vi "Example While Loop Some Operations 2.vi"(8 "Error In":errorcluster, 11 "Boolean":bool) -> (0 "Error Out":errorcluster, 3 "Numeric":i32)   [LabVIEW 2018]
doc: "Testing VI contains WhileLoop and som operations inside and some other constants and functions for numbers used inside WhileLoop. Just for example parsing."
uses:
  <vilib>/measure/NI_MABase.lvlib
panel:
  out "signal out 4":waveform(dbl)
  out "signal out 3":waveform(dbl)
  out "signal out 2":waveform(dbl)
  out "signal out":waveform(dbl)
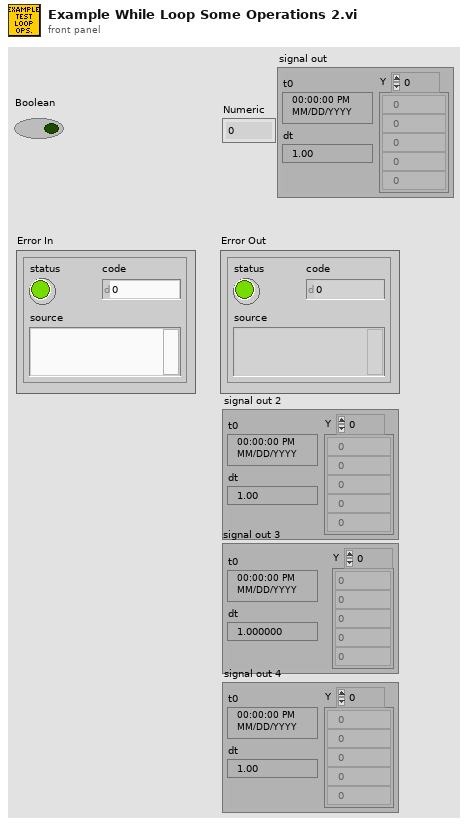
[diagram p1: front panel]
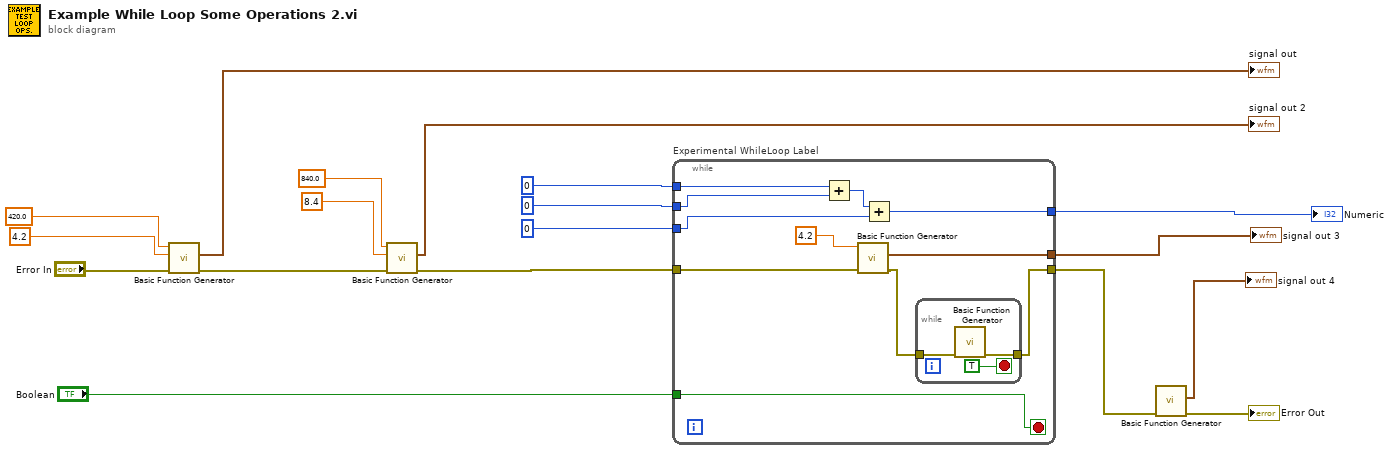
[diagram p0: block diagram]
diagram:
  n1 = call <vilib>:"Basic Function Generator.vi"("error in (no error)"="Error In", "amplitude"=4.2, "frequency"=420.0) -> ("error out"=w12:errorcluster, "signal out"=→"signal out":waveform(dbl))  [unwired: 6 in, 1 out]
  n2 = call <vilib>:"Basic Function Generator.vi"("error in (no error)"=w12, "amplitude"=8.4, "frequency"=840.0) -> ("error out"=w11:errorcluster, "signal out"=→"signal out 2":waveform(dbl))  [unwired: 6 in, 1 out]
  n3 = while "Experimental WhileLoop Label" {
    tunnel: 0 -> [w28]
    tunnel: 0 -> [w27]
    tunnel: 0 -> [w26]
    tunnel: "Boolean" -> [w25]
    tunnel: [w24] -> w14
    tunnel: w11 -> [w23]
    tunnel: [w19] -> w3
    tunnel: [w22] -> w4
    stop <- w25 stop-if-true
    n4 = Add(x=w28, y=w27) -> (x+y=w29:i32)
    n5 = call <vilib>:"Basic Function Generator.vi"("error in (no error)"=w23, "frequency"=4.2) -> ("error out"=w20:errorcluster, "signal out"=w22:waveform(dbl))  [unwired: 7 in, 1 out]
    n6 = Add(x=w29, y=w26) -> (x+y=w24:i32)
    n7 = while {
      tunnel: [w31] -> w19
      tunnel: w20 -> [w32]
      stop <- TRUE stop-if-true
      n8 = call <vilib>:"Basic Function Generator.vi"("error in (no error)"=w32) -> ("error out"=w31:errorcluster)  [unwired: 8 in, 2 out]
    }
  }
  "Numeric" <- w14
  "signal out 3" <- w4
  n9 = call <vilib>:"Basic Function Generator.vi"("error in (no error)"=w3) -> ("error out"=→"Error Out":errorcluster, "signal out"=→"signal out 4":waveform(dbl))  [unwired: 8 in, 1 out]
